vi "SysLog write contstructs.vi"   [LabVIEW 2016]
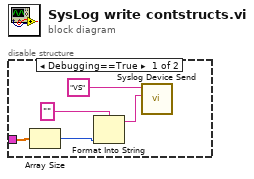
[diagram p0: block diagram]
diagram:
  n1 = disable-structure shown="Debugging==True" {
    disable-tunnel: [w1 w6] -> _
    frame condition #0 (active) {
      n2 = Array Size() -> (array=w1:dbl[], size(s)=w4:i32)
      n3 = Format Into String(format string="", w4) -> (resulting string=w2:string)  [unwired: 2 in, 1 out]
      n4 = call <vilib>:"Syslog Device Send.vi"("Message Content"=w2, "Message Tag"="VS") -> ()  [unwired: 8 in, 2 out]
    }
    frame condition #1 {
    }
  }
